vi "SubVI_SetMeasProp.vi"(8 "error in":errorcluster, 9 "Signal Name":string, 10 "ECU Ref":T1, 11 "XNET Signal In":refnum<k21>) -> (0 "error out":errorcluster, 3 "XNET Signal Out":refnum<k21>)   [LabVIEW 2019, in "XCP_DaqDtoId.lvlib" / "DAQList.lvclass"]
uses:
  DAQList.lvclass
  <vilib>/ECUMC/ECUMC.llb/MC Reference.ctt
  <vilib>/ECUMC/ECUMC.llb/MC Get Prop Meas Comment.vi
  <vilib>/ECUMC/ECUMC.llb/MC Get Prop Meas Scaling Offset.vi
  <vilib>/ECUMC/ECUMC.llb/MC Get Prop Meas Scaling Factor.vi
  <vilib>/ECUMC/ECUMC.llb/MC Get Prop Meas Minimum.vi
  <vilib>/ECUMC/ECUMC.llb/MC Get Prop Meas Maximum.vi
  <vilib>/ECUMC/ECUMC.llb/MC Get Prop Meas Data Type.vi
  <vilib>/ECUMC/ECUMC.llb/MC Get Prop Meas Byte Order.vi
  <vilib>/ECUMC/ECUMC.llb/MC Get Prop Meas Unit.vi
  <resource>/objmgr/xnet.rc
  <vilib>/ECUMC/ECUMC.lvlib
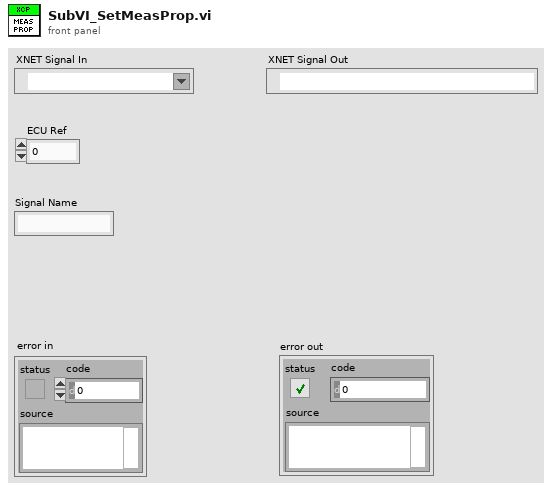
[diagram p1: front panel]
types:
  T1 = typedef "ECUMC.lvlib/MC Reference.ctt" = u32
  T2 = typedef "ECUMC.lvlib/MC Data Type.ctt" = u8
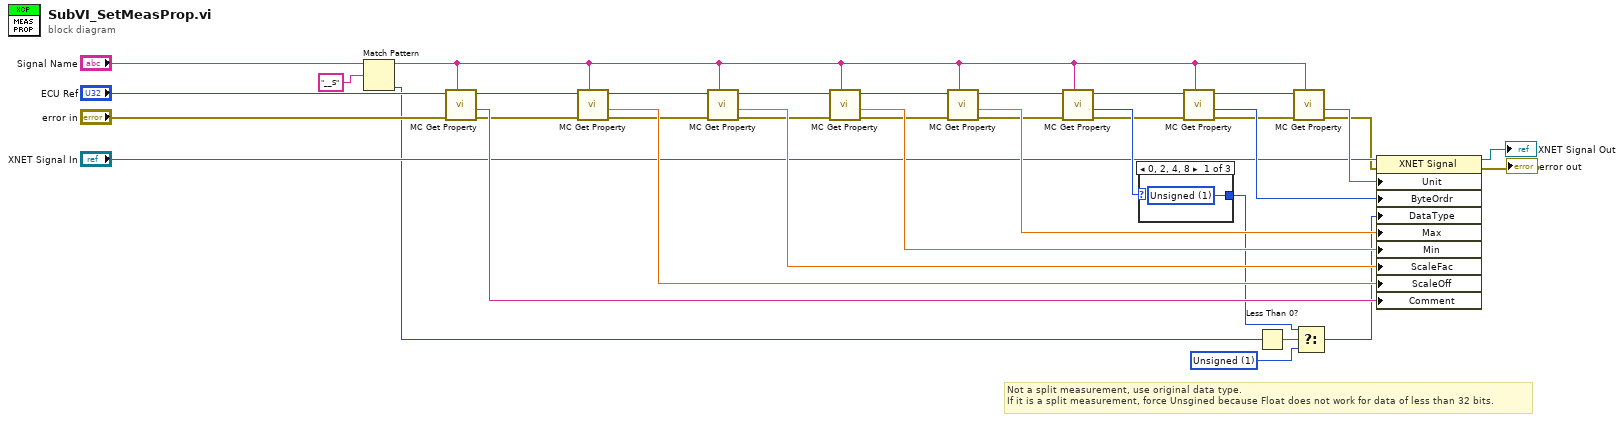
[diagram p0: block diagram]
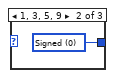
[diagram p2: hidden frame]
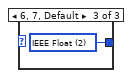
[diagram p3: hidden frame]
diagram:
  w3 = u32 1 items=["Signed", "Unsigned", "IEEE Float", "Byte Array"] ("Data Type")
  # "Not a split measurement, use original data type.\nIf it is a split measurement, force Unsgined because Float does not work for data of less than 32 bits."
  n1 = Match Pattern(string="Signal Name", regular expression="__S") -> (before substring=w5:string, offset past match=w7:i32)  [unwired: 1 in, 2 out]
  n2 = call-poly <vilib>:"MC Get Property.vi"("name"=w5, "error in"="error in", "reference in"="ECU Ref") -> ("error out"=w24:errorcluster, "comment"=w30:string, "reference out"=w25:T1)  [unwired: 6 in]
  n3 = call-poly <vilib>:"MC Get Property.vi"("name"=w5, "error in"=w24, "reference in"=w25) -> ("error out"=w22:errorcluster, "scaling offset"=w31:dbl, "reference out"=w23:T1)  [unwired: 6 in]
  n4 = call-poly <vilib>:"MC Get Property.vi"("name"=w5, "error in"=w22, "reference in"=w23) -> ("error out"=w20:errorcluster, "scaling factor"=w32:dbl, "reference out"=w21:T1)  [unwired: 6 in]
  n5 = call-poly <vilib>:"MC Get Property.vi"("name"=w5, "error in"=w20, "reference in"=w21) -> ("error out"=w18:errorcluster, "meas minimum"=w33:dbl, "reference out"=w19:T1)  [unwired: 6 in]
  n6 = call-poly <vilib>:"MC Get Property.vi"("name"=w5, "error in"=w18, "reference in"=w19) -> ("error out"=w16:errorcluster, "meas maximum"=w34:dbl, "reference out"=w17:T1)  [unwired: 6 in]
  n7 = call-poly <vilib>:"MC Get Property.vi"("name"=w5, "error in"=w16, "reference in"=w17) -> ("error out"=w14:errorcluster, "meas data type"=w29:T2, "reference out"=w15:T1)  [unwired: 6 in]
  n8 = case shown="0, 2, 4, 8" w29 {
    tunnel: [w37 w38 w39] -> w1
    frame 0, 2, 4, 8 {
      w37 = u32 1 items=["Signed", "Unsigned", "IEEE Float", "Byte Array"] ("Data Type")
    }
    frame 1, 3, 5, 9 {
      w38 = u32 0 items=["Signed", "Unsigned", "IEEE Float", "Byte Array"] ("Data Type")
    }
    frame 6, 7, Default {
      w39 = u32 2 items=["Signed", "Unsigned", "IEEE Float", "Byte Array"] ("Data Type")
    }
  }
  n9 = call-poly <vilib>:"MC Get Property.vi"("name"=w5, "error in"=w14, "reference in"=w15) -> ("error out"=w12:errorcluster, "meas byte order"=w35:u32, "reference out"=w13:T1)  [unwired: 6 in]
  n10 = Less Than 0?(x=w7) -> (x < 0?=w4:bool)
  n11 = call-poly <vilib>:"MC Get Property.vi"("name"=w5, "error in"=w12, "reference in"=w13) -> ("error out"=w9:errorcluster, "unit"=w36:string)  [unwired: 6 in, 1 out]
  n12 = Select(t=w1, s=w4, f=w3) -> (s? t:f=w2:u32)
  n13 = property class="XNET Signal"(reference="XNET Signal In", error in=w9, "Unit"=w36, "ByteOrdr"=w35, "DataType"=w2, "Max"=w34, "Min"=w33, "ScaleFac"=w32, "ScaleOff"=w31, "Comment"=w30) -> (reference out=→"XNET Signal Out":refnum<k21>, error out=→"error out":errorcluster)
